vi "ep_D to Y convert (Spectra).vi"(8 "error in (no error)":errorcluster, 10 "line voltage spectra":T2(array[cluster])) -> (0 "error out":errorcluster, 3 "phase voltage spectra":T2(array[cluster]))   [LabVIEW 2014, in "NI_EP_Power Quality.lvlib"]
uses:
  <vilib>/addons/Electrical Power/PQ/NI_EP_Power Quality.lvlib
  <vilib>/addons/Electrical Power/PQ/Common/Controls/ep_AI Data Channel.ctl
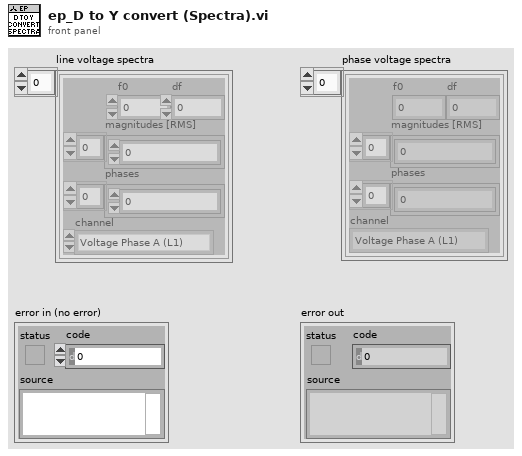
[diagram p1: front panel]
types:
  T1 = typedef "NI_EP_Power Quality.lvlib/ep_AI Data Channel.ctl" = enum16{"Voltage Phase A (L1)", "Voltage Phase B (L2)", "Voltage Phase C (L3)", "Voltage Phase N (Neutral)", "Current Phase A (L1)", "Current Phase B (L2)", "Current Phase C (L3)", "Current Phase N (Neutral)"}
  T2 = cluster{"f0":dbl, "df":dbl, "magnitudes [RMS]":dbl[], "phases":dbl[], "channel":T1}[]
  T3 = cluster{"f0":dbl, "df":dbl, "magnitudes [RMS]":dbl[], "phases":dbl[], "channel":T1}
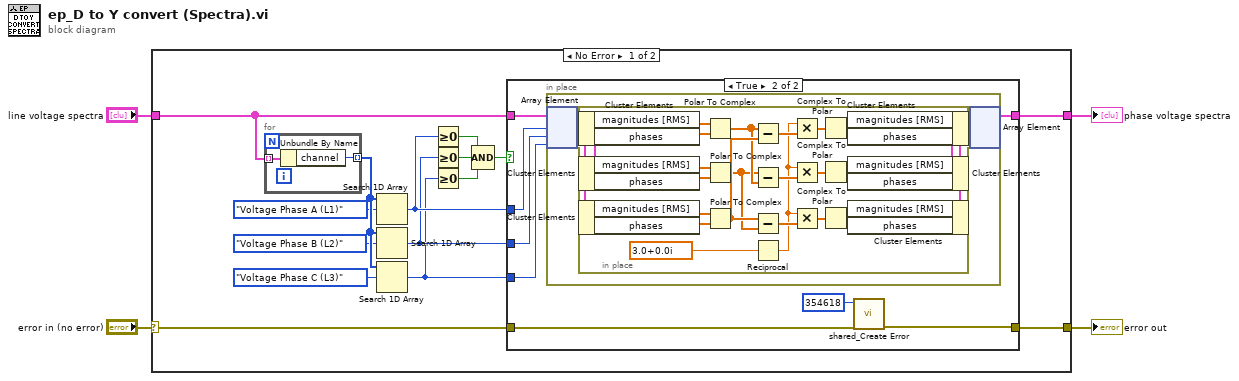
[diagram p0: block diagram]
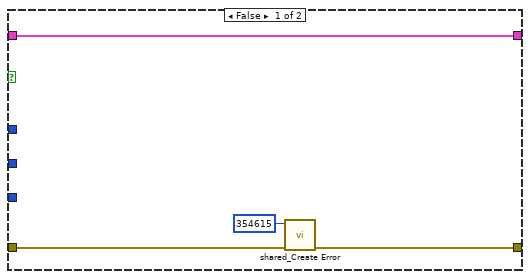
[diagram p2: hidden frame]
diagram:
  n1 = case shown="No Error" "error in (no error)" {
    selector: "error in (no error)" -> [w16 w64]
    tunnel: [w17 w64] -> w3
    tunnel: [w19 w63] -> w2
    tunnel: "line voltage spectra" -> [w18 w63]
    frame No Error {
      n2 = for {
        tunnel: w18 -> [w21] mode=indexing
        tunnel: [w20] -> w13 mode=indexing
        n3 = Unbundle By Name(w21) -> ("channel"=w20:T1)
      }
      n4 = Search 1D Array(1D array=w13, element=ep_AI_Data_Channel."Voltage Phase A (L1)" ("AI data channel")) -> (index of element=w8:i32)  [unwired: 1 in]
      n5 = Search 1D Array(1D array=w13, element=ep_AI_Data_Channel."Voltage Phase B (L2)" ("AI data channel")) -> (index of element=w6:i32)  [unwired: 1 in]
      n6 = Search 1D Array(1D array=w13, element=ep_AI_Data_Channel."Voltage Phase C (L3)" ("AI data channel")) -> (index of element=w5:i32)  [unwired: 1 in]
      n7 = Greater Or Equal To 0?(x=w8) -> (x >= 0?=w9:bool)
      n8 = Greater Or Equal To 0?(x=w6) -> (x >= 0?=w14:bool)
      n9 = Greater Or Equal To 0?(x=w5) -> (x >= 0?=w15:bool)
      n10 = Compound Arithmetic op=AND(w9, w14, w15) -> (w7:bool)
      n11 = case shown="True" w7 {
        tunnel: [w25 w32] -> w19
        tunnel: w18 -> [w25 w33]
        tunnel: w8 -> [_ w31]
        tunnel: w6 -> [_ w30]
        tunnel: w5 -> [_ w29]
        tunnel: w16 -> [w23 w27]
        tunnel: [w22 w26] -> w17
        frame False {
          n12 = call <vilib>:"shared_Create Error.vi"("error in (no error)"=w23, "error code (0)"=354615) -> ("error out"=w22:errorcluster)  [unwired: 9 in]
        }
        frame True {
          n13 = in-place {
            n14 = in-place-array #1(w33, w31, w30, w29) -> (w39:T3, w38:T3, w37:T3)
            n15 = in-place {
              n16 = in-place-cluster #2(w39) -> ("magnitudes [RMS]"=w61:dbl[], "phases"=w62:dbl[])
              n17 = in-place-cluster #3(w38) -> ("magnitudes [RMS]"=w58:dbl[], "phases"=w57:dbl[])
              n18 = in-place-cluster #4(w37) -> ("magnitudes [RMS]"=w55:dbl[], "phases"=w56:dbl[])
              n19 = Polar To Complex(1:w62, 2:w61) -> (0:w48:cdb[])
              n20 = Polar To Complex(1:w57, 2:w58) -> (0:w47:cdb[])
              n21 = Polar To Complex(1:w56, 2:w55) -> (0:w49:cdb[])
              n22 = Subtract(x=w48, y=w49) -> (x-y=w46:cdb[])
              n23 = Subtract(x=w47, y=w48) -> (x-y=w44:cdb[])
              n24 = Subtract(x=w49, y=w47) -> (x-y=w43:cdb[])
              n25 = Reciprocal(x=cdb 3.0+0.0i) -> (1/x=w40:cdb)
              n26 = Multiply(x=w40, y=w46) -> (x*y=w45:cdb[])
              n27 = Multiply(x=w40, y=w44) -> (x*y=w41:cdb[])
              n28 = Multiply(x=w40, y=w43) -> (x*y=w42:cdb[])
              n29 = Complex To Polar(r * e^(i*theta)=w45) -> (r=w60:dbl[], theta=w59:dbl[])
              n30 = Complex To Polar(r * e^(i*theta)=w41) -> (r=w54:dbl[], theta=w53:dbl[])
              n31 = Complex To Polar(r * e^(i*theta)=w42) -> (r=w52:dbl[], theta=w51:dbl[])
              n32 = in-place-cluster #2("magnitudes [RMS]"=w60, "phases"=w59) -> (w36:T3)
              n33 = in-place-cluster #3("magnitudes [RMS]"=w54, "phases"=w53) -> (w35:T3)
              n34 = in-place-cluster #4("magnitudes [RMS]"=w52, "phases"=w51) -> (w34:T3)
            }
            n35 = in-place-array #1(w36, w35, w34) -> (w32:T2)  [unwired: 3 out]
          }
          n36 = call <vilib>:"shared_Create Error.vi"("error in (no error)"=w27, "error code (0)"=354618) -> ("error out"=w26:errorcluster)  [unwired: 9 in]
        }
      }
    }
    frame Error {
    }
  }
  "phase voltage spectra" <- w2
  "error out" <- w3
